vi "unpack projected images.vi"(10 "projected volumes":T2) -> (2 "projections":T1, 4 "zx 2d sizes":i32[](array[numeric]), 5 "zx 1d size":i32)   [LabVIEW 2010]
uses:
  projected_volumes.ctl
  projection buffers.ctl
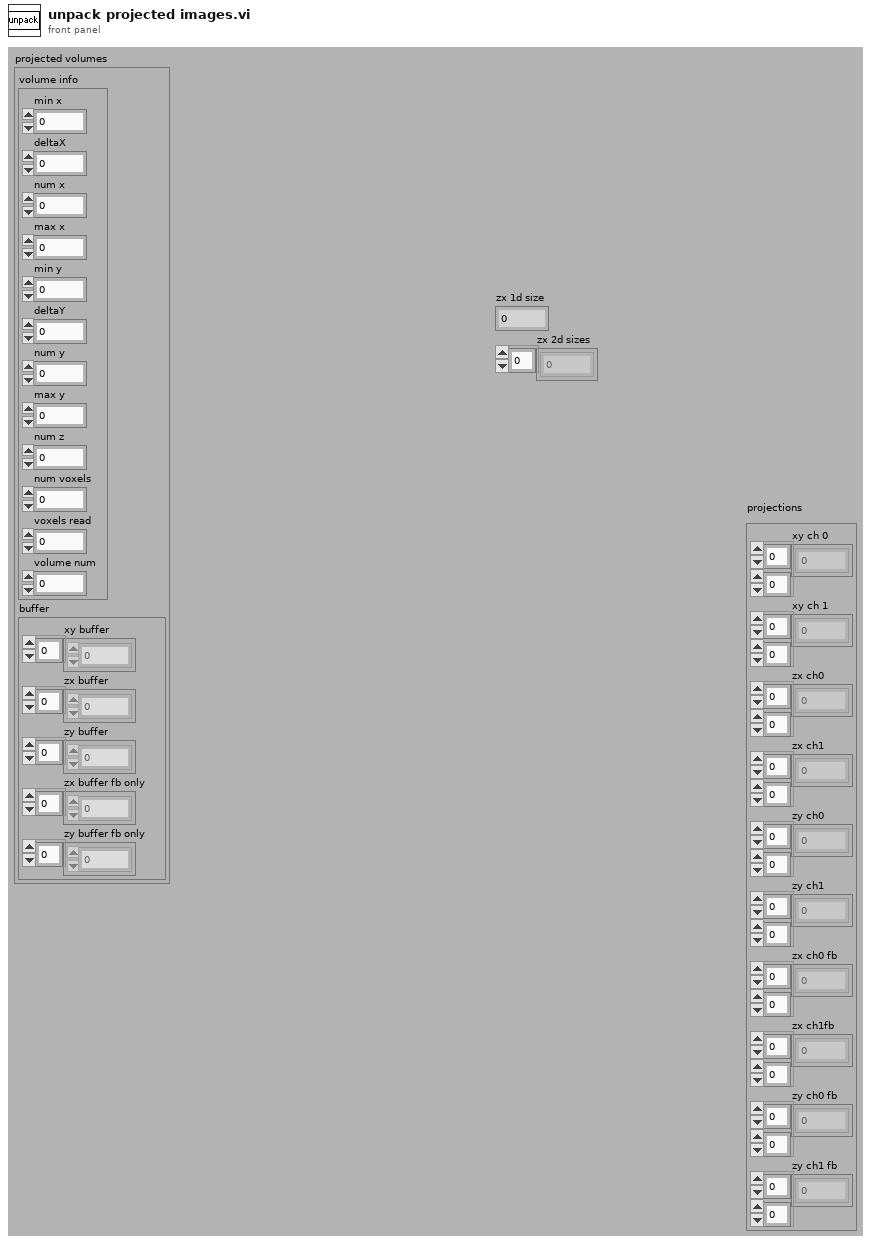
[diagram p1: front panel]
types:
  T1 = cluster{"xy ch 0":dbl[][], "xy ch 1":dbl[][], "zx ch0":dbl[][], "zx ch1":dbl[][], "zy ch0":dbl[][], "zy ch1":dbl[][], "zx ch0 fb":dbl[][], "zx ch1fb":dbl[][], "zy ch0 fb":dbl[][], "zy ch1 fb":dbl[][]}
  T2 = typedef "projected_volumes.ctl" = cluster{"volume info":cluster{"min x":i16, "deltaX":dbl, "num x":u32, "max x":i16, "min y":i16, "deltaY":dbl, "num y":u32, "max y":i16, "num z":u32, "num voxels":u32, "voxels read":u32, "volume num":u32}, "buffer":T3}
  T3 = typedef "projection buffers.ctl" = cluster{"xy buffer":u32[], "zx buffer":u32[], "zy buffer":u32[], "zx buffer fb only":u32[], "zy buffer fb only":u32[]}
  T4 = cluster{"xy ch 0":u16[][], "xy ch 1":u16[][], "zx ch0":u16[][], "zx ch1":u16[][], "zy ch0":u16[][], "zy ch1":u16[][], "zx ch0 fb":u16[][], "zx ch1fb":u16[][], "zy ch0 fb":u16[][], "zy ch1 fb":u16[][]}
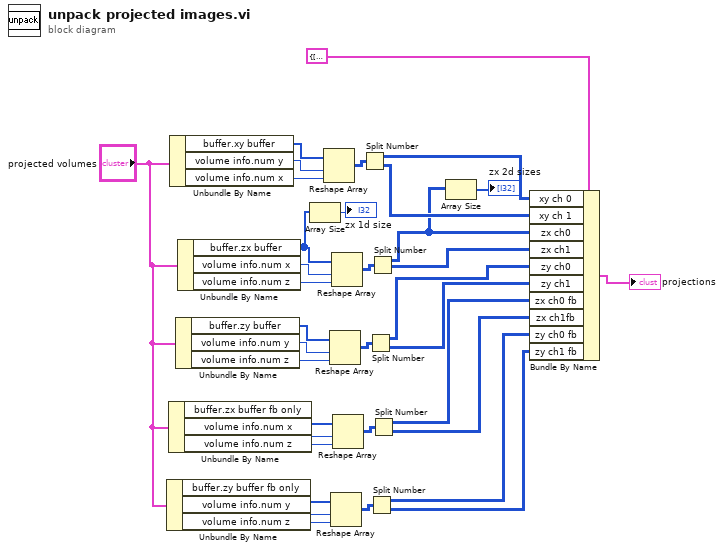
[diagram p0: block diagram]
diagram:
  n1 = Unbundle By Name("projected volumes") -> ("buffer.zy buffer fb only"=w20:u32[], "volume info.num y"=w19:u32, "volume info.num z"=w18:u32)
  n2 = Unbundle By Name("projected volumes") -> ("buffer.zx buffer fb only"=w24:u32[], "volume info.num x"=w23:u32, "volume info.num z"=w22:u32)
  n3 = Unbundle By Name("projected volumes") -> ("buffer.xy buffer"=w35:u32[], "volume info.num y"=w34:u32, "volume info.num x"=w33:u32)
  n4 = Unbundle By Name("projected volumes") -> ("buffer.zy buffer"=w28:u32[], "volume info.num y"=w27:u32, "volume info.num z"=w26:u32)
  n5 = Unbundle By Name("projected volumes") -> ("buffer.zx buffer"=w4:u32[], "volume info.num x"=w31:u32, "volume info.num z"=w30:u32)
  n6 = Array Size(array=w4) -> (size(s)=→"zx 1d size":i32)
  n7 = Reshape Array(w35, w34, w33) -> (w32:u32[][])
  n8 = Reshape Array(w28, w27, w26) -> (w25:u32[][])
  n9 = Reshape Array(w20, w19, w18) -> (w17:u32[][])
  n10 = Reshape Array(w4, w31, w30) -> (w29:u32[][])
  n11 = Reshape Array(w24, w23, w22) -> (w21:u32[][])
  n12 = Split Number(x=w32) -> (hi(x)=w14:u16[][], lo(x)=w13:u16[][])
  n13 = Split Number(x=w25) -> (hi(x)=w11:u16[][], lo(x)=w10:u16[][])
  n14 = Split Number(x=w17) -> (hi(x)=w7:u16[][], lo(x)=w6:u16[][])
  n15 = Split Number(x=w29) -> (hi(x)=w2:u16[][], lo(x)=w12:u16[][])
  n16 = Split Number(x=w21) -> (hi(x)=w9:u16[][], lo(x)=w8:u16[][])
  n17 = Array Size(array=w2) -> (size(s)=→"zx 2d sizes":i32[])
  n18 = Bundle By Name(cluster=T4 {"xy ch 0"=[], "xy ch 1"=[], "zx ch0"=[], "zx ch1"=[], "zy ch0"=[], "zy ch1"=[], "zx ch0 fb"=[], "zx ch1fb"=[], "zy ch0 fb"=[], "zy ch1 fb"=[]} ("projections"), "xy ch 0"=w14, "xy ch 1"=w13, "zx ch0"=w2, "zx ch1"=w12, "zy ch0"=w11, "zy ch1"=w10, "zx ch0 fb"=w9, "zx ch1fb"=w8, "zy ch0 fb"=w7, "zy ch1 fb"=w6) -> (→"projections":T4)
